vi "Final ATM machine.vi"() -> ()   [LabVIEW 2020]
uses:
  control 3.ctl
panel:
  out "collect cash":string
  out "blink":string
  out "Denomination":string
  in  "Amount entry btn":bool
  in  "Numeric amount":i32=100 min=100 max=100000 step=100
  out "Insert ATM card":string
  in  "PIn btn":bool
  in  "PIN String":string
  in  "Enter user name 2":bool
  in  "Username 2":string
  out "Info string":string
  in  "Insert card 2":bool
  out "Welcome 2":string
  in  "Cancel 1":bool
  in  "Home 2":bool
  in  "Enter Password":bool
  in  "Password":string
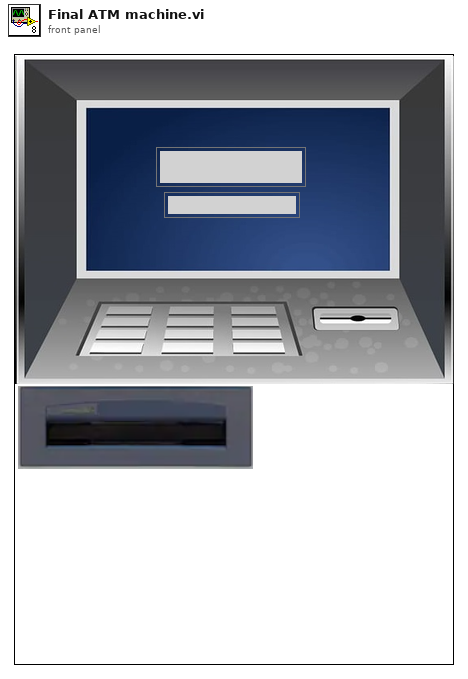
[diagram p1: front panel]
types:
  T1 = typedef "control 3.ctl" = enum16{"initialize", "Amount page", "Welcome page", "Thank You", "enable amt num", "display amount", "abort", "Wait after thank you", "Enter amount page"}
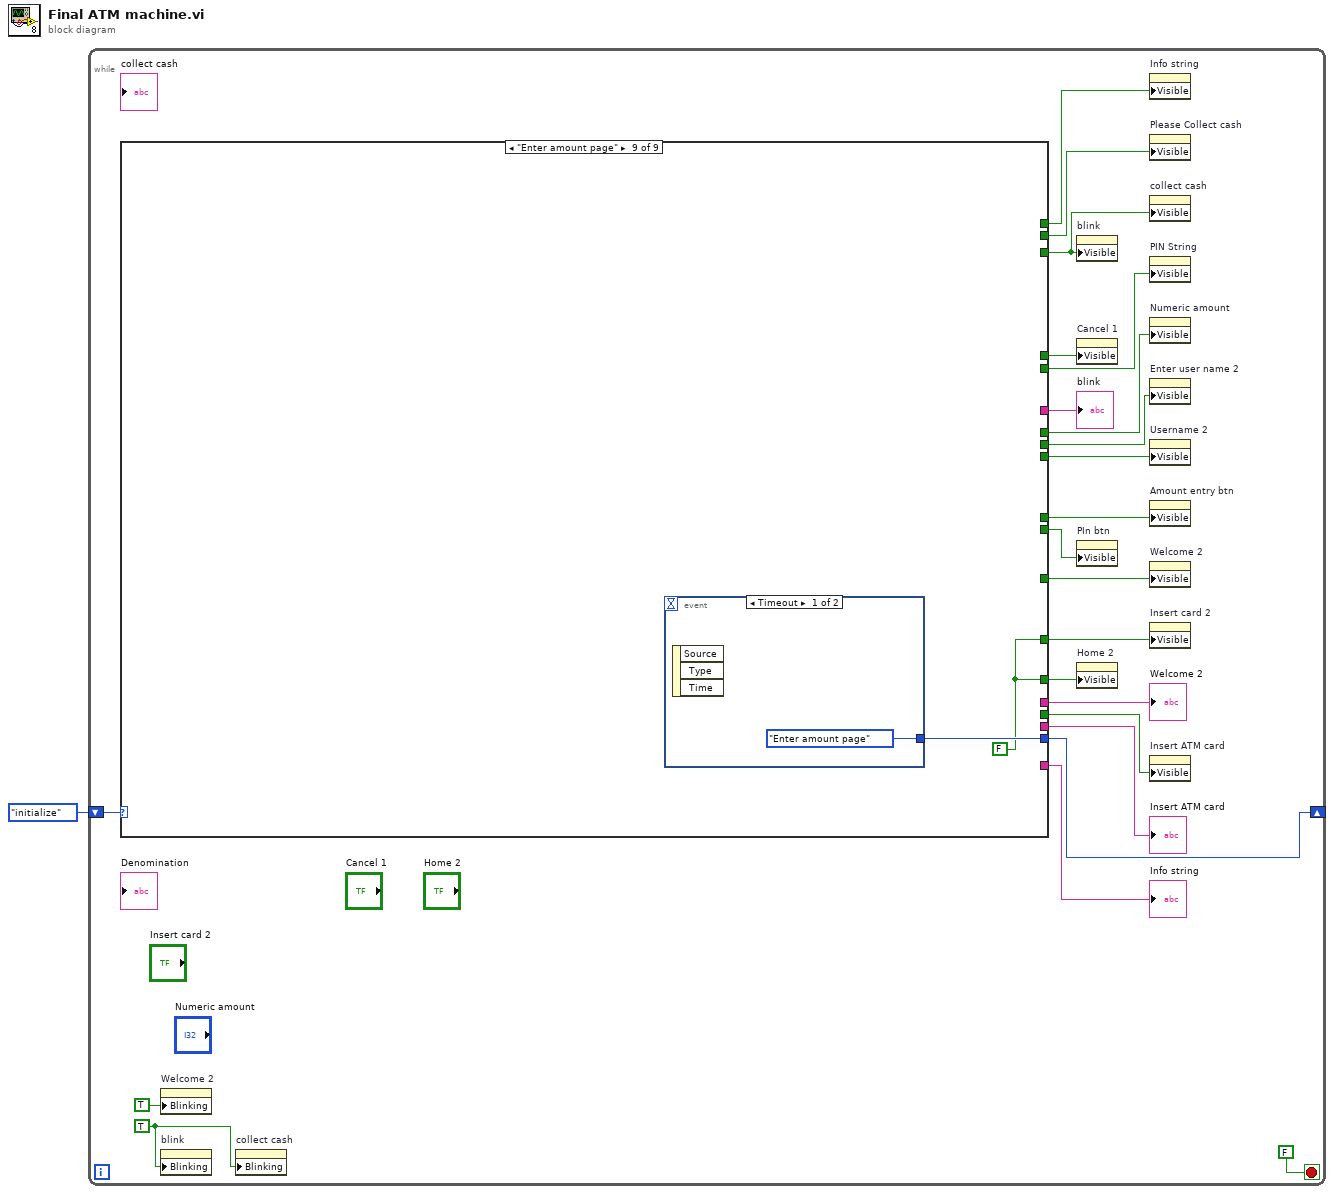
[diagram p0: block diagram]
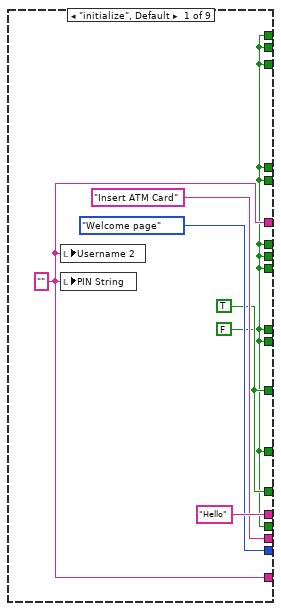
[diagram p2: hidden frame]
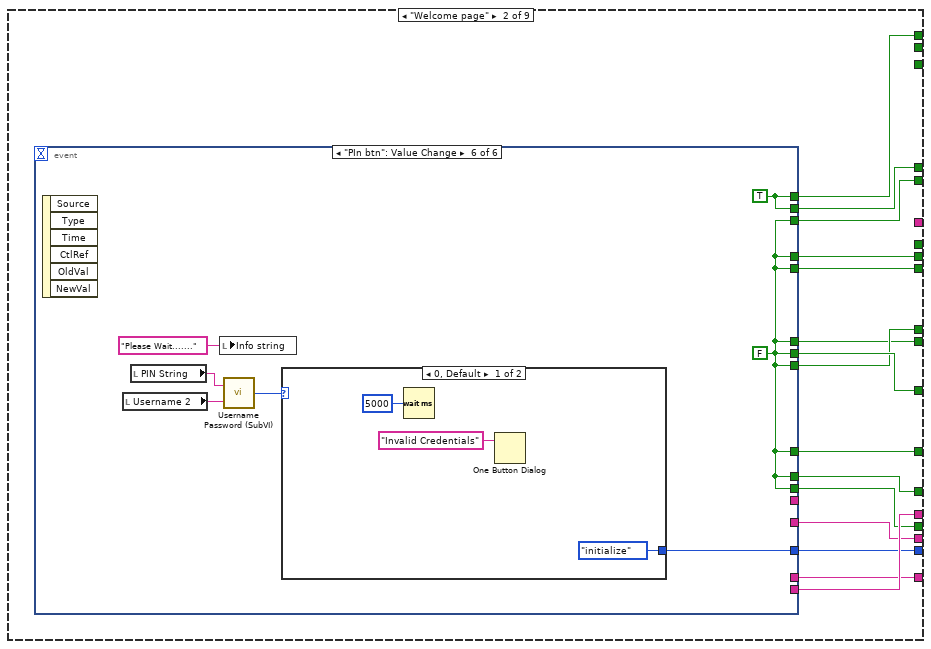
[diagram p3: hidden frame]
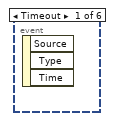
[diagram p4: hidden frame]
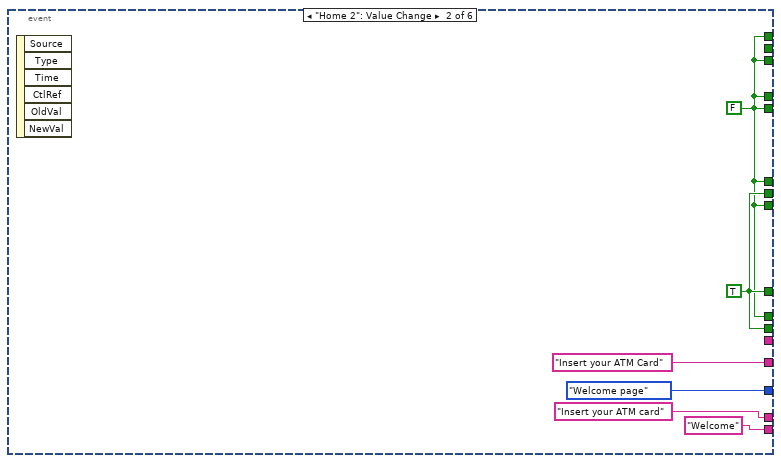
[diagram p5: hidden frame]
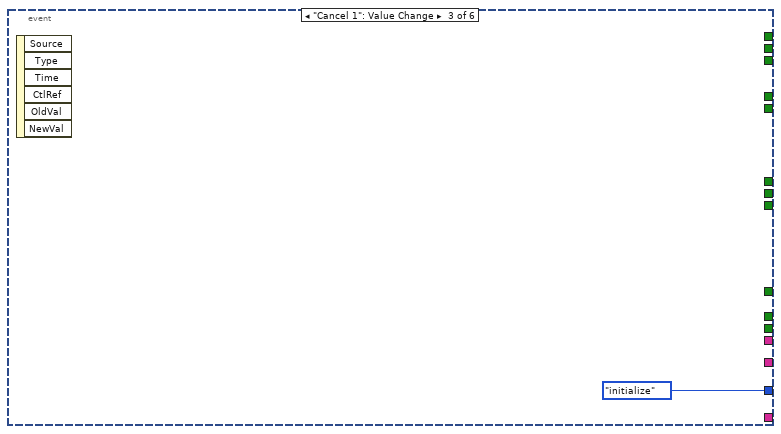
[diagram p6: hidden frame]
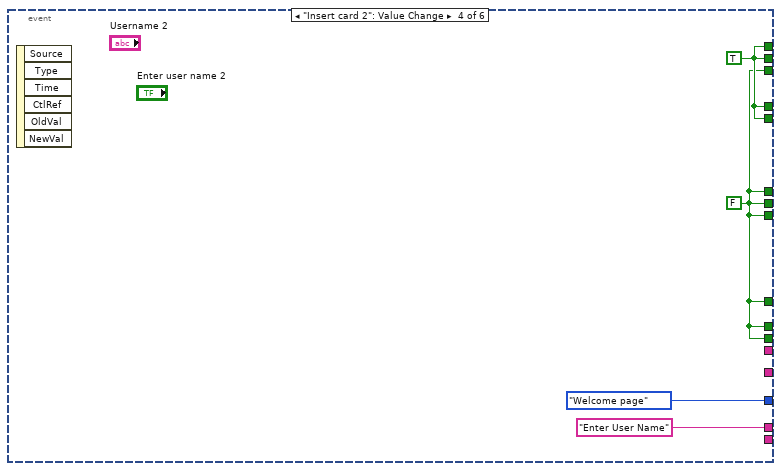
[diagram p7: hidden frame]
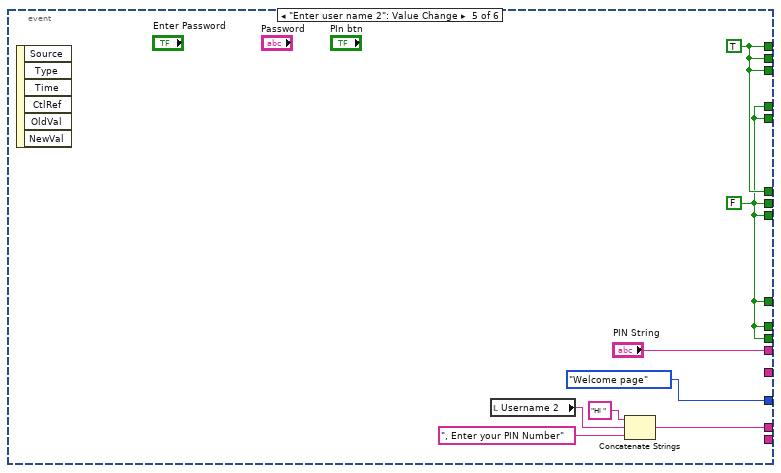
[diagram p8: hidden frame]
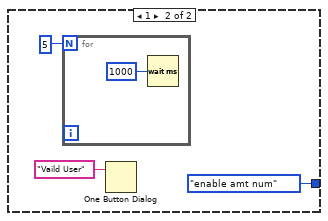
[diagram p9: hidden frame]
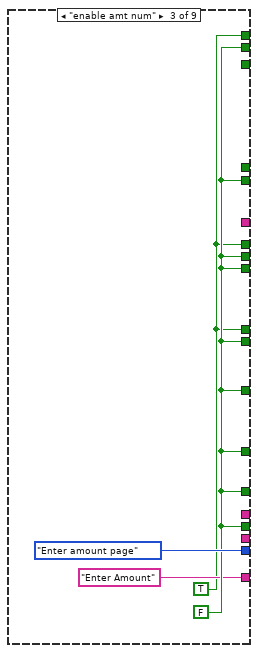
[diagram p10: hidden frame]
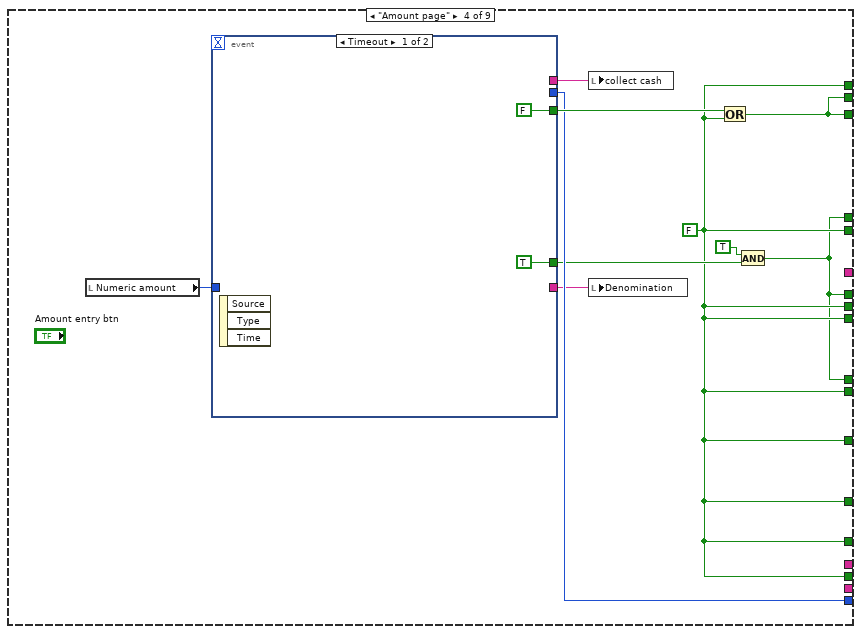
[diagram p11: hidden frame]
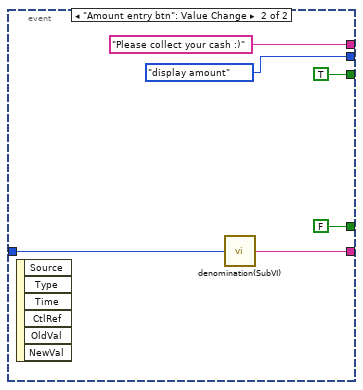
[diagram p12: hidden frame]
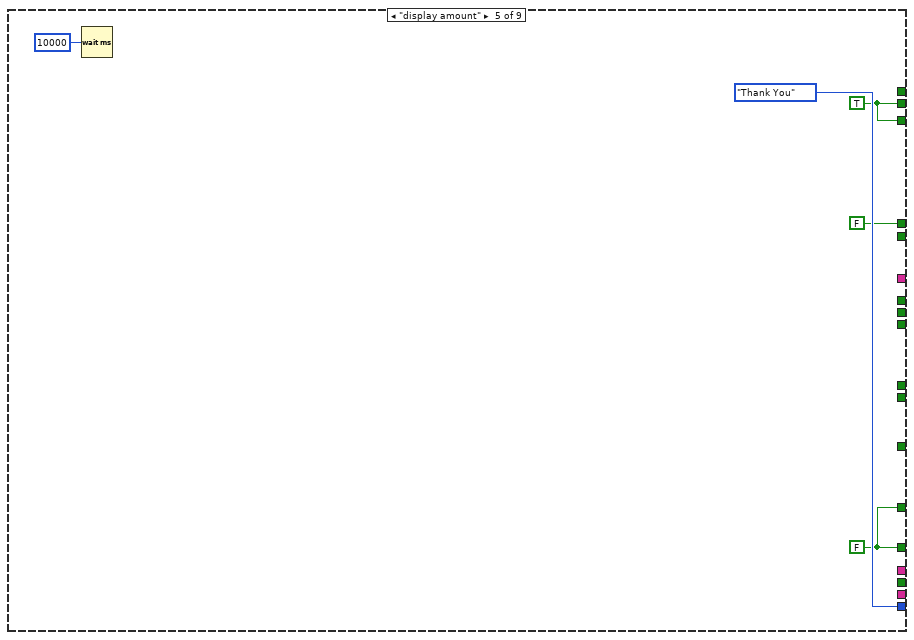
[diagram p13: hidden frame]
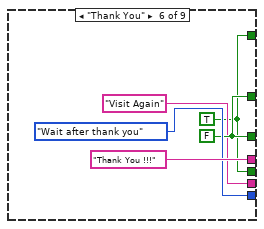
[diagram p14: hidden frame]
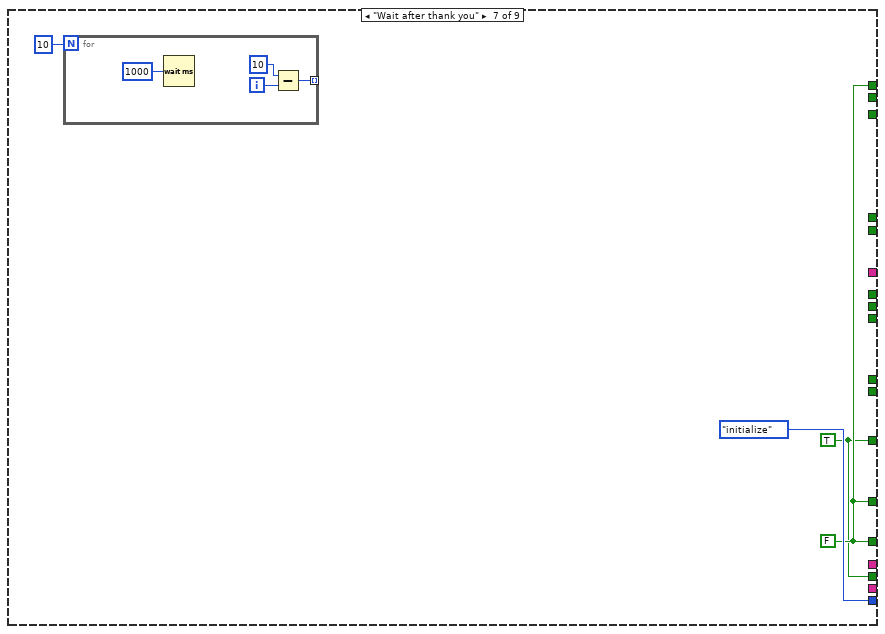
[diagram p15: hidden frame]
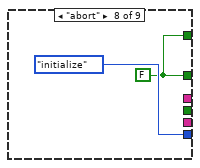
[diagram p16: hidden frame]
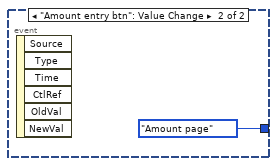
[diagram p17: hidden frame]
diagram:
  n1 = while {
    shift-right: [w23] -> _
    shift-left: control_3."initialize" -> [w22]
    stop <- FALSE stop-if-true
    w2 = TRUE ("Blinking")
    n2 = case shown="\"Enter amount page\"" w22 {
      tunnel: ["Hello" w45 _ _ _ "Thank You !!!" _ _ _] -> w19
      tunnel: ["Insert ATM Card" w41 _ _ _ "Visit Again" _ _ _] -> w9
      tunnel: [w27 w42 w81 w89 _ w106 w111 _ _] -> w18
      tunnel: [w25 w40 w81 w89 _ w106 w111 _ _] -> w8
      tunnel: [w25 w44 w81 w89 _ _ _ _ _] -> w13
      tunnel: [w25 w43 w81 w89 _ _ _ _ _] -> w11
      tunnel: [control_3."Welcome page" w39 control_3."Enter amount page" w91 control_3."Thank You" control_3."Wait after thank you" control_3."initialize" control_3."initialize" w122] -> w23
      tunnel: [w25 w34 w81 w89 _ _ _ _ _] -> w12
      tunnel: [w25 w35 w81 w89 _ _ _ _ _] -> w10
      tunnel: [w25 w36 w79 w86 _ _ _ _ _] -> w6
      tunnel: [w26 w38 "Enter Amount" _ _ _ _ _ _] -> w15
      tunnel: [w25 w37 w79 w89 _ _ w112 _ _] -> w14
      tunnel: [w25 _ w79 w86 _ _ _ _ _] -> w7
      tunnel: [w25 _ w81 w84 w101 _ _ _ _] -> w5
      tunnel: [w25 w32 w81 w89 w104 w108 w112 w119 w121] -> w17
      tunnel: [w27 w33 w81 w89 w104 w108 w112 w119 w121] -> w20
      tunnel: [w25 w31 _ w86 FALSE _ _ _ _] -> w21
      tunnel: [w26 _ _ _ _ _ _ _ _] -> w4
      tunnel: [w25 _ _ w84 w101 _ _ _ _] -> w3
      frame "initialize", Default {
        w25 = FALSE
        w27 = TRUE
        w26 = ""
        n3 = local write "Username 2"(w26) -> ()
        n4 = local write "PIN String"(w26) -> ()
      }
      frame "Welcome page" {
        n5 = event shown="[5] \"PIn btn\": Value Change" {
          selector: _ -> [_ _ _ _ _ _]
          dyn-events: _ -> [_ _ _ _ _ _]
          timeout: _ -> [_ _ _ _ _ _]
          tunnel: [_ "Welcome" _ _ _ _] -> w45
          tunnel: [_ w47 _ w54 w59 w68] -> w44
          tunnel: [_ w47 _ w53 w60 w68] -> w43
          tunnel: [_ w48 _ w53 w59 w68] -> w42
          tunnel: [_ w48 _ w53 w59 w68] -> w40
          tunnel: [_ "Insert your ATM Card" _ _ _ _] -> w41
          tunnel: [_ control_3."Welcome page" control_3."initialize" control_3."Welcome page" control_3."Welcome page" w70] -> w39
          tunnel: [_ "Insert your ATM card" _ "Enter User Name" w64 _] -> w38
          tunnel: [_ w47 _ w54 w60 w69] -> w37
          tunnel: [_ w47 _ w53 w59 w68] -> w36
          tunnel: [_ w47 _ w53 w60 w68] -> w35
          tunnel: [_ w47 _ w54 w59 w68] -> w34
          tunnel: [_ _ _ _ "PIN String" _] -> _
          tunnel: [_ w47 _ w53 w59 w68] -> w33
          tunnel: [_ w48 _ w53 w59 w68] -> w32
          tunnel: [_ _ _ w54 w60 w69] -> w31
          event Timeout {
            n6 = event-data() -> ()  [unwired: 1 in, 3 out]
          }
          event "Home 2": Value Change {
            w48 = TRUE
            w47 = FALSE
            n7 = event-data() -> ()  [unwired: 1 in, 6 out]
          }
          event "Cancel 1": Value Change {
            n8 = event-data() -> ()  [unwired: 1 in, 6 out]
          }
          event "Insert card 2": Value Change {
            w54 = TRUE
            w53 = FALSE
            n9 = event-data() -> ()  [unwired: 1 in, 6 out]
          }
          event "Enter user name 2": Value Change {
            w59 = FALSE
            w60 = TRUE
            n10 = event-data() -> ()  [unwired: 1 in, 6 out]
            n11 = local read "Username 2"() -> (w58:string)
            n12 = Concatenate Strings("Hi " ("string"), w58, ", Enter your PIN Number" ("string")) -> (w64:string)
          }
          event "PIn btn": Value Change {
            w68 = FALSE
            w69 = TRUE
            n13 = event-data() -> ()  [unwired: 1 in, 6 out]
            n14 = local read "Username 2"() -> (w67:string)
            n15 = local read "PIN String"() -> (w66:string)
            n16 = local write "Info string"("Please Wait.......") -> ()
            n17 = call "Username Password (SubVI).vi"("Username"=w67, "Password"=w66) -> ("0, 1"=w71:i16)
            n18 = case shown="0, Default" w71 {
              tunnel: [control_3."initialize" control_3."enable amt num"] -> w70
              frame 0, Default {
                n19 = Wait (ms)(milliseconds to wait=u32 5000) -> ()  [unwired: 1 out]
                n20 = One Button Dialog(message="Invalid Credentials") -> ()  [unwired: 1 in, 1 out]
              }
              frame 1 {
                n21 = for {
                  N: 5 -> [_]
                  n22 = Wait (ms)(milliseconds to wait=u32 1000) -> ()  [unwired: 1 out]
                }
                n23 = One Button Dialog(message="Vaild User") -> ()  [unwired: 1 in, 1 out]
              }
            }
          }
        }
      }
      frame "enable amt num" {
        w79 = TRUE
        w81 = FALSE
      }
      frame "Amount page" {
        w89 = FALSE
        n24 = local read "Numeric amount"() -> (w85:i32)
        n25 = event shown="[0] Timeout" {
          selector: _ -> [_ _]
          dyn-events: _ -> [_ _]
          timeout: _ -> [_ _]
          tunnel: [_ w100] -> w87
          tunnel: [FALSE TRUE] -> w92
          tunnel: [_ control_3."display amount"] -> w91
          tunnel: w85 -> [_ w96]
          tunnel: [TRUE FALSE] -> w90
          tunnel: [_ "Please collect your cash :)"] -> w83
          event Timeout {
            n26 = event-data() -> ()  [unwired: 1 in, 3 out]
          }
          event "Amount entry btn": Value Change {
            n27 = event-data() -> ()  [unwired: 1 in, 6 out]
            n28 = call "denomination(SubVI).vi"("Enter Amount"=w96) -> ("String"=w100:string)
          }
        }
        n29 = local write "collect cash"(w83) -> ()
        n30 = local write "Denomination"(w87) -> ()
        n31 = Or(x=w92, y=w89) -> (x .or. y?=w84:bool)
        n32 = And(x=TRUE, y=w90) -> (x .and. y?=w86:bool)
      }
      frame "display amount" {
        w101 = TRUE
        w104 = FALSE
        n33 = Wait (ms)(milliseconds to wait=u32 10000) -> ()  [unwired: 1 out]
      }
      frame "Thank You" {
        w108 = FALSE
        w106 = TRUE
      }
      frame "Wait after thank you" {
        w111 = TRUE
        w112 = FALSE
        n34 = for {
          N: 10 -> [_]
          tunnel: [w115] -> _ mode=indexing
          i -> [w116]
          n35 = Wait (ms)(milliseconds to wait=u32 1000) -> ()  [unwired: 1 out]
          n36 = Subtract(x=10, y=w116) -> (x-y=w115:i32)
        }
      }
      frame "abort" {
        w119 = FALSE
      }
      frame "Enter amount page" {
        w121 = FALSE
        n37 = event shown="[0] Timeout" {
          selector: _ -> [_ _]
          dyn-events: _ -> [_ _]
          timeout: _ -> [_ _]
          tunnel: [control_3."Enter amount page" control_3."Amount page"] -> w122
          event Timeout {
            n38 = event-data() -> ()  [unwired: 1 in, 3 out]
          }
          event "Amount entry btn": Value Change {
            n39 = event-data() -> ()  [unwired: 1 in, 6 out]
          }
        }
      }
    }
    "Welcome 2" <- w19
    "Info string" <- w15
    "Insert ATM card" <- w9
    "blink" <- w4
    n40 = property on="Welcome 2" class="Str"("Blinking"=TRUE) -> ()  [unwired: 2 in, 2 out]
    n41 = property on="blink" class="Str"("Blinking"=w2) -> ()  [unwired: 2 in, 2 out]
    n42 = property on="collect cash" class="Str"("Blinking"=w2) -> ()  [unwired: 2 in, 2 out]
    n43 = property on="blink" class="Str"("Visible"=w3) -> ()  [unwired: 2 in, 2 out]
    n44 = property on="Cancel 1" class="Bool"("Visible"=w21) -> ()  [unwired: 2 in, 2 out]
    n45 = property on="PIn btn" class="Bool"("Visible"=w10) -> ()  [unwired: 2 in, 2 out]
    n46 = property on="Home 2" class="Bool"("Visible"=w20) -> ()  [unwired: 2 in, 2 out]
    n47 = property on="Info string" class="Str"("Visible"=w14) -> ()  [unwired: 2 in, 2 out]
    n48 = property on="Please Collect cash" class="Str"("Visible"=w5) -> ()  [unwired: 2 in, 2 out]
    n49 = property on="collect cash" class="Str"("Visible"=w3) -> ()  [unwired: 2 in, 2 out]
    n50 = property on="PIN String" class="Str"("Visible"=w11) -> ()  [unwired: 2 in, 2 out]
    n51 = property on="Numeric amount" class="DigNum (strict)"("Visible"=w7) -> ()  [unwired: 2 in, 2 out]
    n52 = property on="Enter user name 2" class="Bool"("Visible"=w12) -> ()  [unwired: 2 in, 2 out]
    n53 = property on="Username 2" class="Str"("Visible"=w13) -> ()  [unwired: 2 in, 2 out]
    n54 = property on="Amount entry btn" class="Bool"("Visible"=w6) -> ()  [unwired: 2 in, 2 out]
    n55 = property on="Welcome 2" class="Str"("Visible"=w18) -> ()  [unwired: 2 in, 2 out]
    n56 = property on="Insert card 2" class="Bool"("Visible"=w17) -> ()  [unwired: 2 in, 2 out]
    n57 = property on="Insert ATM card" class="Str"("Visible"=w8) -> ()  [unwired: 2 in, 2 out]
  }
